vi "Basic Correction Setup.vi"(0 "VISA resource name":refnum<visa-resource-name>, 1 "Load Corr  (F: Off)":bool, 2 "Short Corr (T: On)":bool=TRUE, 3 "Open Corr  (F: Off)":bool, 5 "Cable Length (0: 4 m)":u32(slide)=4 max=4, 7 "Corr Method (T: Single)":bool=TRUE, 9 "Load Type (0: CPD)":u32(ring) items=["CPD", "CPQ", "CPG", "CPRP", "CSD", "CSQ", "CSRS", "LPQ", "LPD", "LPG", "LPRP", "LSD", "LSQ", "LSRS", "RX", "ZTD", "ZTR", "GB", "YTD", "YTR"], 11 "error in (no error)":errorcluster, 12 "Channel Num (0)":i16 min=0 max=89 step=1) -> (4 "VISA resource name out":refnum<visa-resource-name>, 8 "Tmo Value":u32, 15 "error out":errorcluster)   [LabVIEW 2015, in "Agilent 428X Series.lvlib"]
doc: "This function sets the cable length settings, and the OPEN/SHORT/LOAD correction settings."
uses:
  Agilent 428X Series.lvlib
panel:
  # "On\nOff"
  # "On\nOff"
  # "On\nOff"
  # "Single\nMulti"
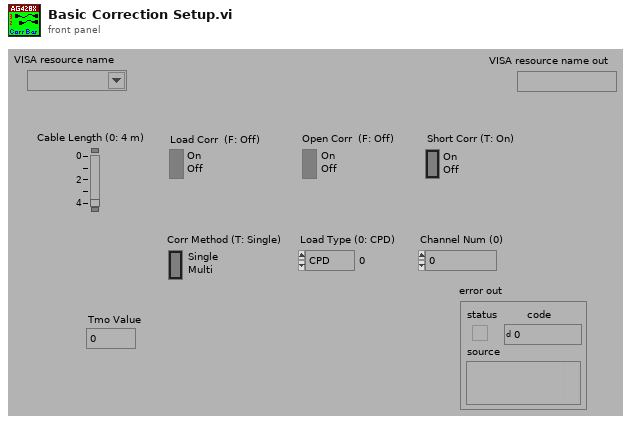
[diagram p1: front panel]
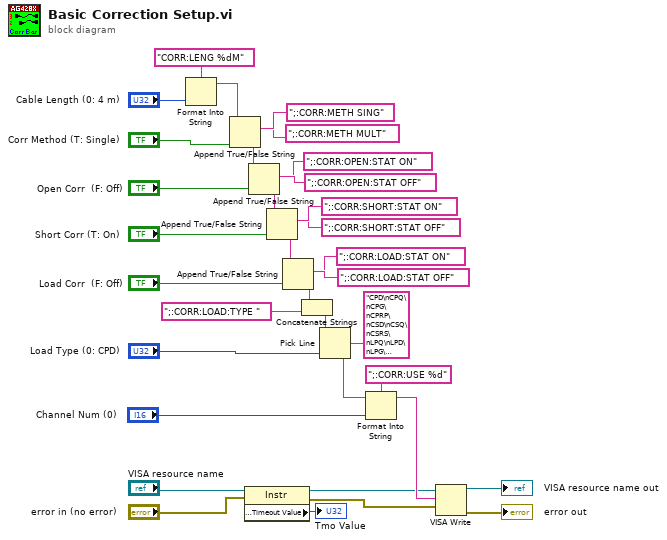
[diagram p0: block diagram]
diagram:
  n1 = Format Into String(format string="CORR:LENG %dM", "Cable Length (0: 4 m)") -> (resulting string=w31:string)  [unwired: 2 in, 1 out]
  n2 = Append True/False String(1:"Corr Method (T: Single)", 2:";:CORR:METH MULT" ("true string"), 3:";:CORR:METH SING" ("true string"), 4:w31) -> (0:w27:string)
  n3 = property class="Instr"(reference="VISA resource name", error in="error in (no error)") -> (reference out=w3:refnum<visa-resource-name>, error out=w2:errorcluster, "General Settings:Timeout Value"=→"Tmo Value":u32)
  n4 = Append True/False String(1:"Open Corr  (F: Off)", 2:";:CORR:OPEN:STAT OFF", 3:";:CORR:OPEN:STAT ON", 4:w27) -> (0:w20:string)
  n5 = Append True/False String(1:"Short Corr (T: On)", 2:";:CORR:SHORT:STAT OFF", 3:";:CORR:SHORT:STAT ON", 4:w20) -> (0:w19:string)
  n6 = Append True/False String(1:"Load Corr  (F: Off)", 2:";:CORR:LOAD:STAT OFF", 3:";:CORR:LOAD:STAT ON", 4:w19) -> (0:w16:string)
  n7 = Concatenate Strings(w16, ";:CORR:LOAD:TYPE ") -> (w14:string)
  n8 = Pick Line(string ("")=w14, multi-line string="CPD\nCPQ\nCPG\nCPRP\nCSD\nCSQ\nCSRS\nLPQ\nLPD\nLPG\nLPRP\nLSD\nLSQ\nLSRS\nRX\nZTD\nZTR\nGB\nYTD\nYTR", line index="Load Type (0: CPD)") -> (output string=w10:string)
  n9 = Format Into String(format string=";:CORR:USE %d", initial string=w10, "Channel Num (0)") -> (resulting string=w6:string)  [unwired: 1 in, 1 out]
  n10 = VISA Write(VISA resource name=w3, write buffer=w6, error in (no error)=w2) -> (VISA resource name out=→"VISA resource name out":refnum<visa-resource-name>, error out=→"error out":errorcluster)  [unwired: 1 out]
